vi "New In Range Trigger.vi"(8 "error in (no error)":errorcluster, 9 "Invert":bool, 10 "Lower Limit":dbl, 11 "Upper Limit":dbl) -> (0 "error out":errorcluster, 3 "In Range Trigger out":refnum<class "In Range Trigger.lvclass">)   [LabVIEW 2012, in "Waveform Data Logger Engine.lvlib" / "In Range Trigger.lvclass"]
uses:
  In Range Trigger.lvclass
  In Range Trigger.lvclass/In Range Trigger.ctl
  Trigger/Trigger Type.ctl
  Trigger/Trigger.lvclass/Trigger.ctl
  Trigger/Write Trigger Type.vi
  Trigger/Trigger.lvclass
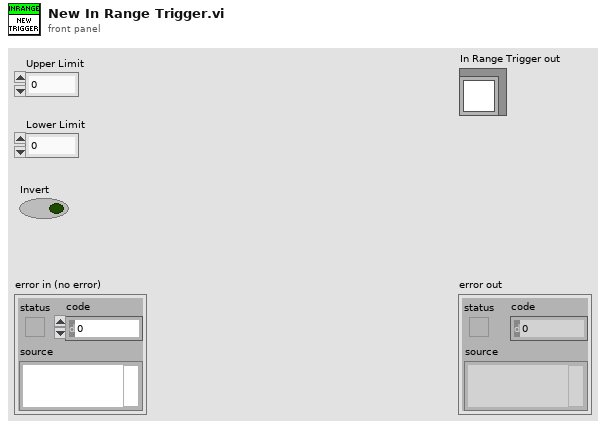
[diagram p1: front panel]
types:
  T1 = typedef "Waveform Data Logger Engine.lvlib/Trigger.lvclass/Trigger Type.ctl" = enum16{"Default", "Digital Edge", "Analog Edge", "In Range", "Value Change", "Boolean Evaluation"}
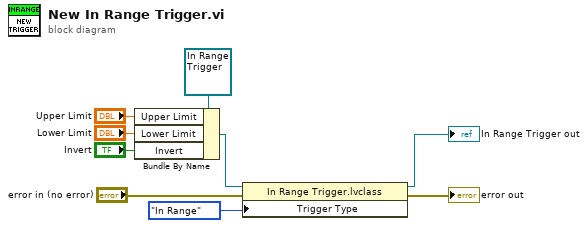
[diagram p0: block diagram]
diagram:
  n1 = Bundle By Name(cluster=refnum<class "In Range Trigger.lvclass"> refnum ("In Range Trigger in"), "Upper Limit"="Upper Limit", "Lower Limit"="Lower Limit", "Invert"="Invert") -> (w3:refnum<class "In Range Trigger.lvclass">)
  n2 = property class="In Range Trigger.lvclass"(reference=w3, error in="error in (no error)", "Trigger Type"=Trigger_Type."In Range") -> (reference out=→"In Range Trigger out":refnum<class "In Range Trigger.lvclass">, error out=→"error out":errorcluster)
